vi "Query Limit Test Results.vi"(8 "error in (no error)":errorcluster, 11 "VISA resource name":refnum<visa-resource-name>) -> (0 "error out":errorcluster, 1 "Failure Number (0)":i32, 2 "Pass Number (0)":i32, 3 "VISA resource name out":refnum<visa-resource-name>, 5 "Total Number (0)":i32)   [LabVIEW 2012, in "Tektronix TDS 200 1000 2000 Series.lvlib"]
doc: "This VI queries the limit test results."
uses:
  <instrlib>/Tektronix TDS 200 1000 2000 Series/Tektronix TDS 200 1000 2000 Series.lvlib
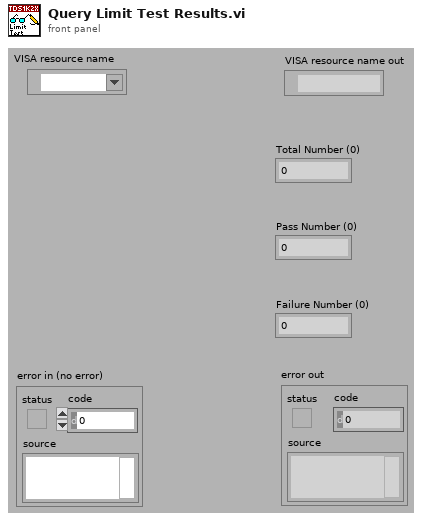
[diagram p1: front panel]
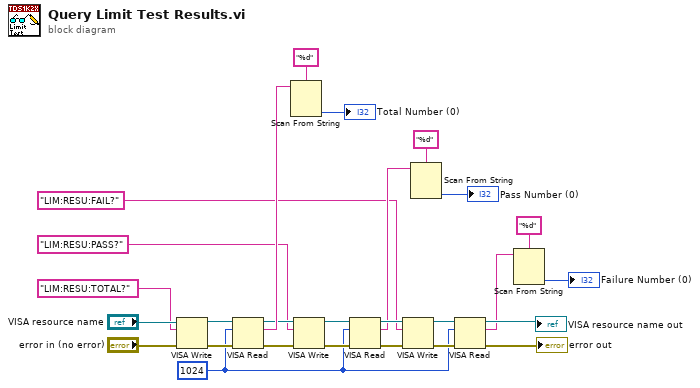
[diagram p0: block diagram]
diagram:
  w6 = u32 1024 ("byte count")
  n1 = VISA Write(VISA resource name="VISA resource name", write buffer="LIM:RESU:TOTAL?", error in (no error)="error in (no error)") -> (VISA resource name out=w25:refnum<visa-resource-name>, error out=w26:errorcluster)  [unwired: 1 out]
  n2 = VISA Read(VISA resource name=w25, byte count=w6, error in (no error)=w26) -> (VISA resource name out=w17:refnum<visa-resource-name>, read buffer=w23:string, error out=w16:errorcluster)  [unwired: 1 out]
  n3 = Scan From String(format string="%d", input string=w23) -> (output 1=→"Total Number (0)":i32)  [unwired: 2 in, 4 out]
  n4 = VISA Write(VISA resource name=w17, write buffer="LIM:RESU:PASS?", error in (no error)=w16) -> (VISA resource name out=w20:refnum<visa-resource-name>, error out=w21:errorcluster)  [unwired: 1 out]
  n5 = VISA Read(VISA resource name=w20, byte count=w6, error in (no error)=w21) -> (VISA resource name out=w15:refnum<visa-resource-name>, read buffer=w10:string, error out=w14:errorcluster)  [unwired: 1 out]
  n6 = VISA Write(VISA resource name=w15, write buffer="LIM:RESU:FAIL?", error in (no error)=w14) -> (VISA resource name out=w18:refnum<visa-resource-name>, error out=w19:errorcluster)  [unwired: 1 out]
  n7 = Scan From String(format string="%d", input string=w10) -> (output 1=→"Pass Number (0)":i32)  [unwired: 2 in, 4 out]
  n8 = VISA Read(VISA resource name=w18, byte count=w6, error in (no error)=w19) -> (VISA resource name out=→"VISA resource name out":refnum<visa-resource-name>, read buffer=w9:string, error out=→"error out":errorcluster)  [unwired: 1 out]
  n9 = Scan From String(format string="%d", input string=w9) -> (output 1=→"Failure Number (0)":i32)  [unwired: 2 in, 4 out]
